vi "test Compile RaF Channel Data.vi"(8 "error in (no error)":errorcluster, 11 "TestCase in":refnum<class "Routing and Faulting Compile Unit Tests.lvclass">) -> (0 "error out":errorcluster, 3 "TestCase out":refnum<class "Routing and Faulting Compile Unit Tests.lvclass">)   [LabVIEW 2017, in "Routing and Faulting Compile Unit Tests.lvclass"]
uses:
  Routing and Faulting Compile Unit Tests.lvclass
  Shared/Communication Configuration.ctl
  Shared/Routing and Faulting Configuration.ctl
  Shared/Routing Channel Configuration.ctl
  Shared/Value-Connections Map.ctl
  Shared/Connection.ctl
  Shared/Alias Mapping.ctl
  Shared/FIFO Indices.ctl
  Shared/Channel States.ctl
  Shared/Routing State.ctl
  Shared/Compiled.Settings.ctl
  Routing and Faulting Compile Unit Tests.lvclass/Routing and Faulting Compile Unit Tests.ctl
  System Explorer/Get Channel Data in By Channel ID (offline).vi
  Scripting/Switch Scripting.lvlib
  Shared/Routing and Faulting Shared.lvlib
  System Explorer/Routing and Faulting System Explorer.lvlib
panel:
  out "Compiled.Settings":T8
  in  "Save?":bool
  out "Output Filename":string
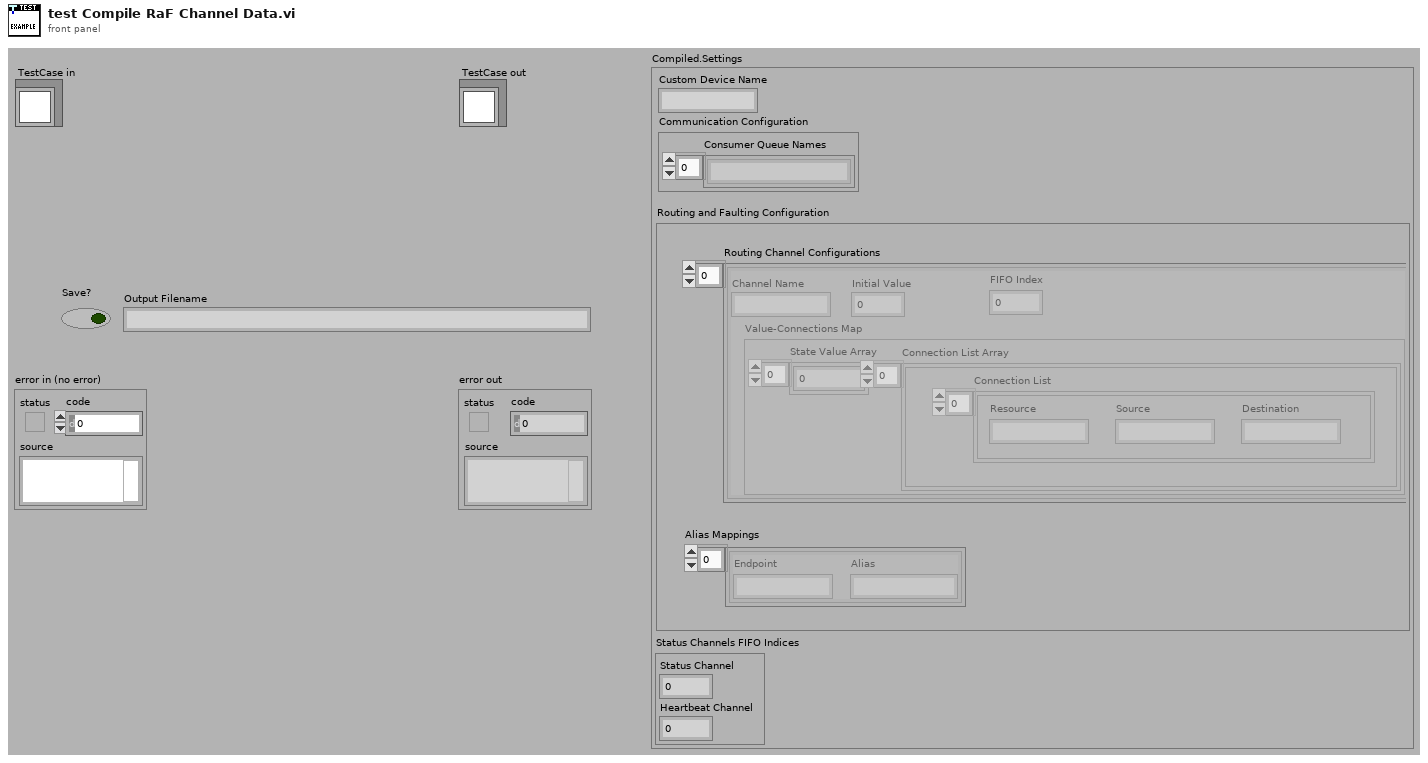
[diagram p1: front panel]
types:
  T1 = typedef "Routing and Faulting Shared.lvlib/Communication Configuration.ctl" = cluster{"Consumer Queue Names":string[]}
  T2 = typedef "Routing and Faulting Shared.lvlib/Routing and Faulting Configuration.ctl" = cluster{"Routing Channel Configurations":T3[], "Alias Mappings":T6[]}
  T3 = typedef "Routing and Faulting Shared.lvlib/Routing Channel Configuration.ctl" = cluster{"Channel Name":string, "Initial Value":dbl, "FIFO Index":i32, "Value-Connections Map":T4}
  T4 = typedef "Routing and Faulting Shared.lvlib/Value-Connections Map.ctl" = cluster{"State Value Array":i32[], "Connection List Array":cluster{"Connection List":T5[]}[]}
  T5 = typedef "Routing and Faulting Shared.lvlib/Connection.ctl" = cluster{"Resource":string, "Source":string, "Destination":string}
  T6 = typedef "Routing and Faulting Shared.lvlib/Alias Mapping.ctl" = cluster{"Endpoint":string, "Alias":string}
  T7 = typedef "Routing and Faulting Shared.lvlib/FIFO Indices.ctl" = cluster{"Status Channel":i32, "Heartbeat Channel":i32}
  T8 = cluster{"Custom Device Name":string, "Communication Configuration":T1, "Routing and Faulting Configuration":T2, "Status Channels FIFO Indices":T7}
  T9 = typedef "Routing and Faulting Shared.lvlib/Compiled.Settings.ctl" = cluster{"Custom Device Name":string, "Communication Configuration":T1, "Routing and Faulting Configuration":T2, "Status Channels FIFO Indices":T7}
  T10 = typedef "Routing and Faulting Shared.lvlib/Channel States.ctl" = T11[]
  T11 = typedef "Routing and Faulting Shared.lvlib/Routing State.ctl" = cluster{"Name":string, "Description":string, "Value":i32, "Connection List":T5[]}
  T12 = typedef "Custom Device API.lvlib/Custom Device Item Ref.ctl" = u64
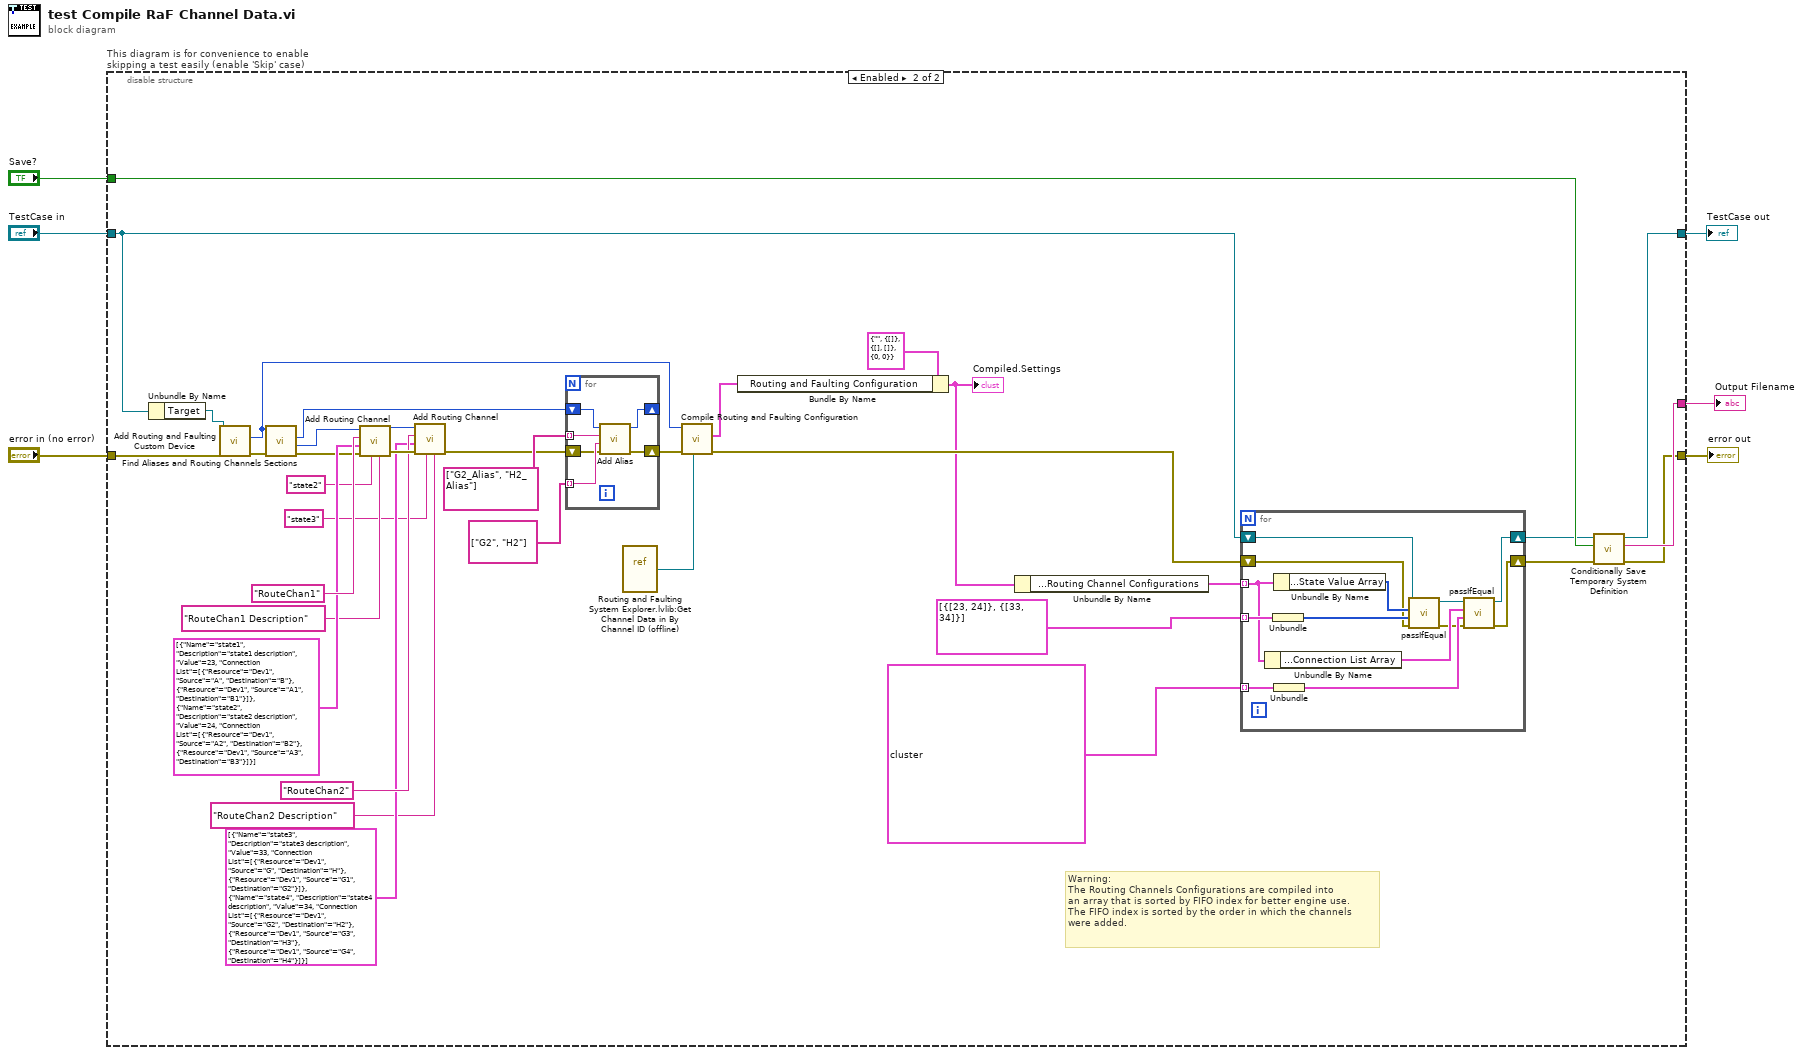
[diagram p0: block diagram]
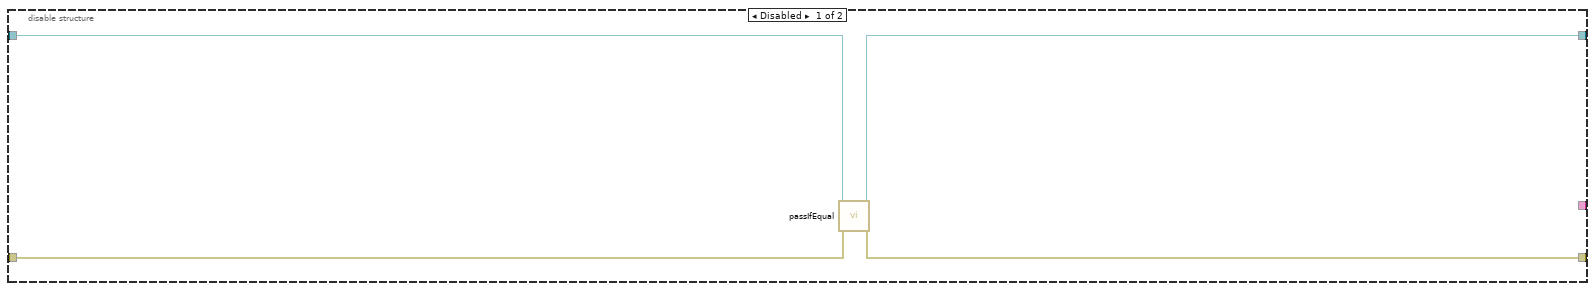
[diagram p2: hidden frame]
diagram:
  n1 = disable-structure "This diagram is for convenience to enable skipping a test easily (enable 'Skip' case)" shown="Enabled" {
    disable-tunnel: "TestCase in" -> [w10 w36]
    disable-tunnel: [w9 w41] -> w3
    disable-tunnel: [w8 w30] -> w5
    disable-tunnel: "error in (no error)" -> [w7 w43]
    disable-tunnel: "Save?" -> [_ w42]
    disable-tunnel: [_ w40] -> w1
    frame Disabled {
      n2 = call-dynamic "passIfEqual.vi"("error in (no error)"=w7, "TestCase in"=w10) -> ("error out"=w8:errorcluster, "TestCase out"=w9:refnum<class "Routing and Faulting Compile Unit Tests.lvclass">)  [unwired: 8 in]
    }
    frame Enabled {
      # "Warning: \nThe Routing Channels Configurations are compiled into\nan array that is sorted by FIFO index for better engine use.\nThe FIFO index is sorted by the order in which the channels\nwere added."
      n3 = Unbundle By Name(w36) -> ("Target"=w44:refnum<k24>)
      n4 = call "Add Routing and Faulting Custom Device.vi"("error in (no error)"=w43, "Target in"=w44) -> ("error out"=w46:errorcluster, "Routing and Faulting Custom Device Ref"=w14:T12)  [unwired: 7 in, 1 out]
      n5 = call "Find Aliases and Routing Channels Sections.vi"("error in (no error)"=w46, "Routing and Faulting Custom Device Ref in"=w14) -> ("error out"=w24:errorcluster, "Routing Channels Ref"=w23:T12, "Aliases Ref"=w22:T12)  [unwired: 6 in, 1 out]
      n6 = call "Add Routing Channel.vi"("Description"="RouteChan1 Description", "Initial State"="state2", "error in (no error)"=w24, "State and Connections List"=T10 [{"Name"="state1", "Description"="state1 description", "Value"=23, "Connection List"=[{"Resource"="Dev1", "Source"="A", "Destination"="B"}, {"Resource"="Dev1", "Source"="A1", "Destination"="B1"}]}, {"Name"="state2", "Description"="state2 description", "Value"=24, "Connection List"=[{"Resource"="Dev1", "Source"="A2", "Destination"="B2"}, {"Resource"="Dev1", "Source"="A3", "Destination"="B3"}]}] ("States and Connections"), "Channel Name"="RouteChan1", "Routing Channels Ref in"=w23) -> ("error out"=w39:errorcluster, "Routing Channels Ref out"=w38:T12)  [unwired: 3 in, 1 out]
      n7 = call "Add Routing Channel.vi"("Description"="RouteChan2 Description", "Initial State"="state3", "error in (no error)"=w39, "State and Connections List"=T10 [{"Name"="state3", "Description"="state3 description", "Value"=33, "Connection List"=[{"Resource"="Dev1", "Source"="G", "Destination"="H"}, {"Resource"="Dev1", "Source"="G1", "Destination"="G2"}]}, {"Name"="state4", "Description"="state4 description", "Value"=34, "Connection List"=[{"Resource"="Dev1", "Source"="G2", "Destination"="H2"}, {"Resource"="Dev1", "Source"="G3", "Destination"="H3"}, {"Resource"="Dev1", "Source"="G4", "Destination"="H4"}]}] ("States and Connections"), "Channel Name"="RouteChan2", "Routing Channels Ref in"=w38) -> ("error out"=w26:errorcluster)  [unwired: 3 in, 2 out]
      n8 = for {
        shift-right: [w49] -> _
        shift-left: w22 -> [w50]
        tunnel: string[] ["G2_Alias", "H2_Alias"] -> [w52] mode=indexing
        tunnel: string[] ["G2", "H2"] -> [w51] mode=indexing
        shift-right: [w48] -> w13
        shift-left: w26 -> [w47]
        n9 = call "Add Alias.vi"("error in (no error)"=w47, "Endpoint"=w51, "Alias"=w52, "Aliases Ref in"=w50) -> ("error out"=w48:errorcluster, "Aliases Ref out"=w49:T12)  [unwired: 6 in]
      }
      n10 = vi-ref "Routing and Faulting System Explorer.lvlib:Get Channel Data in By Channel ID (offline).vi"() -> (w11:refnum<vi>)
      n11 = call "Compile Routing and Faulting Configuration.vi"("Get Channel Data Refnum"=w11, "error in (no error)"=w13, "Device Ref in"=w14) -> ("error out"=w16:errorcluster, "RaF Configuration"=w15:T2)  [unwired: 6 in, 1 out]
      n12 = Bundle By Name(cluster=T9 {"Custom Device Name"="", "Communication Configuration"={"Consumer Queue Names"=[]}, "Routing and Faulting Configuration"={"Routing Channel Configurations"=[], "Alias Mappings"=[]}, "Status Channels FIFO Indices"={"Status Channel"=0, "Heartbeat Channel"=0}} ("Compiled.Settings.ctl"), "Routing and Faulting Configuration"=w15) -> (w12:T9)
      "Compiled.Settings" <- w12
      n13 = Unbundle By Name(w12) -> ("Routing and Faulting Configuration.Routing Channel Configurations"=w35:T3[])
      n14 = for {
        tunnel: w35 -> [w59] mode=indexing
        tunnel: cluster{i32[]}[] [{[23, 24]}, {[33, 34]}] ("expected State Values") -> [w65] mode=indexing
        tunnel: cluster{cluster{"Connection List":T5[]}[]}[] [{[{"Connection List"=[{"Resource"="Dev1", "Source"="A", "Destination"="B"}, {"Resource"="Dev1", "Source"="A1", "Destination"="B1"}]}, {"Connection List"=[{"Resource"="Dev1", "Source"="A2", "Destination"="B2"}, {"Resource"="Dev1", "Source"="A3", "Destination"="B3"}]}]}, {[{"Connection List"=[{"Resource"="Dev1", "Source"="G", "Destination"="H"}, {"Resource"="Dev1", "Source"="G1", "Destination"="G2"}]}, {"Connection List"=[{"Resource"="Dev1", "Source"="G2", "Destination"="H2"}, {"Resource"="Dev1", "Source"="G3", "Destination"="H3"}, {"Resource"="Dev1", "Source"="G4", "Destination"="H4"}]}]}] ("expected Connection List data") -> [w61] mode=indexing
        shift-right: [w56] -> w31
        shift-left: w36 -> [w55]
        shift-right: [w53] -> w29
        shift-left: w16 -> [w54]
        n15 = Unbundle By Name(w59) -> ("Value-Connections Map.Connection List Array"=w62:cluster{"Connection List":T5[]}[])
        n16 = Unbundle(w65) -> (w64:i32[])
        n17 = Unbundle By Name(w59) -> ("Value-Connections Map.State Value Array"=w63:i32[])
        n18 = Unbundle(w61) -> (w60:cluster{"Connection List":T5[]}[])
        n19 = call-dynamic "passIfEqual.vi"("error in (no error)"=w54, "y"=w64, "x"=w63, "TestCase in"=w55) -> ("error out"=w58:errorcluster, "TestCase out"=w57:refnum<class "Routing and Faulting Compile Unit Tests.lvclass">)  [unwired: 6 in]
        n20 = call-dynamic "passIfEqual.vi"("error in (no error)"=w58, "y"=w60, "x"=w62, "TestCase in"=w57) -> ("error out"=w53:errorcluster, "TestCase out"=w56:refnum<class "Routing and Faulting Compile Unit Tests.lvclass">)  [unwired: 6 in]
      }
      n21 = call "Conditionally Save Temporary System Definition.vi"("error in (no error)"=w29, "Save?"=w42, "TestCase in"=w31) -> ("error out"=w30:errorcluster, "filename"=w40:string, "TestCase out"=w41:refnum<class "Routing and Faulting Compile Unit Tests.lvclass">)  [unwired: 6 in]
    }
  }
  "error out" <- w5
  "TestCase out" <- w3
  "Output Filename" <- w1
